vi "launch_auto2_test M.vi"(8 "error in (no error)":errorcluster, 10 "modbusData":refnum<notifier>, 11 "Cluster":T1) -> (0 "error out":errorcluster)   [LabVIEW 2019]
uses:
  core_dataRefCluster.ctl
  core_dataRef.ctl
  core_dataCluster.ctl
  instrument/instr_dataCluster.ctl
  instrument/Instrument.lvclass
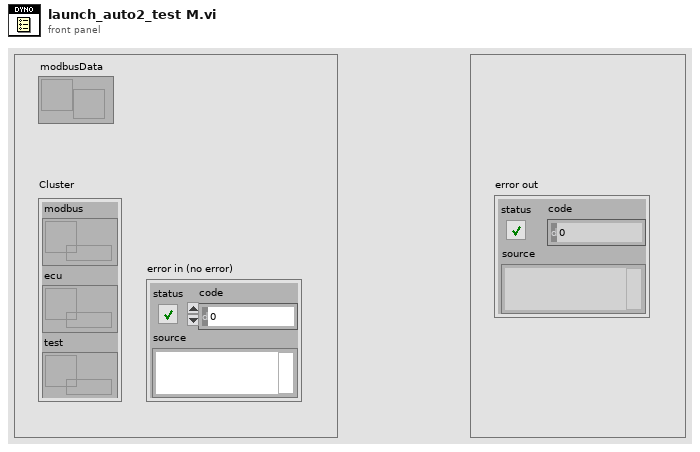
[diagram p1: front panel]
types:
  T1 = typedef "core_dataRefCluster.ctl" = cluster{"modbus":T2, "ecu":T2, "test":T2}
  T2 = typedef "core_dataRef.ctl" = refnum<queue>
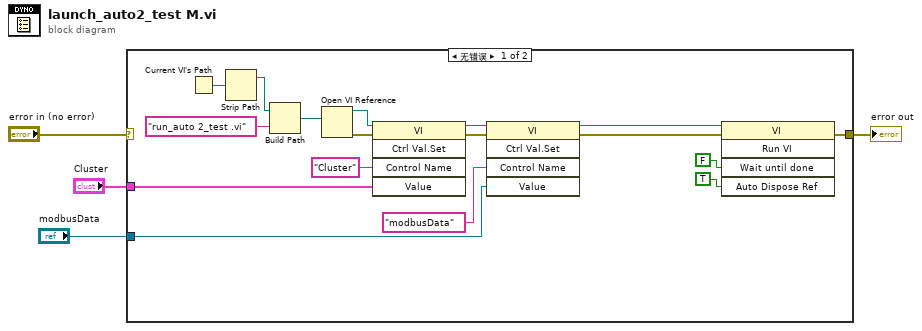
[diagram p0: block diagram]
diagram:
  n1 = case shown="无错误" "error in (no error)" {
    selector: "error in (no error)" -> [_ w22]
    tunnel: "Cluster" -> [w19 _]
    tunnel: "modbusData" -> [w18 _]
    tunnel: [w8 w22] -> w2
    frame No Error {
      n2 = Current VI's Path() -> (path=w15:path)
      n3 = Strip Path(path=w15) -> (stripped path=w14:path)  [unwired: 1 out]
      n4 = Build Path(base path=w14, name or relative path="run_auto 2_test .vi") -> (appended path=w13:path)
      n5 = Open VI Reference(vi path=w13) -> (vi reference=w21:refnum<vi>, error out=w16:errorcluster)  [unwired: 5 in]
      n6 = invoke class="VI" method="Ctrl Val.Set"(reference=w21, error in=w16, "Control Name"="Cluster", "Value"=w19) -> (reference out=w20:refnum<vi>, error out=w17:errorcluster)  [unwired: 1 in, 3 out]
      n7 = invoke class="VI" method="Ctrl Val.Set"(reference=w20, error in=w17, "Control Name"="modbusData", "Value"=w18) -> (reference out=w5:refnum<vi>, error out=w6:errorcluster)  [unwired: 1 in, 3 out]
      n8 = invoke class="VI" method="Run VI"(reference=w5, error in=w6, "Wait until done"=FALSE ("Wait Until Done"), "Auto Dispose Ref"=TRUE ("Auto Dispose Reference")) -> (error out=w8:errorcluster)  [unwired: 1 in, 4 out]
    }
    frame Error {
    }
  }
  "error out" <- w2
